vi "BeginService (reference).vi"(1 "In":i32) -> (0 "Out":i32)   [LabVIEW 2011]
doc: "Copyright (c) 2005, Kuan Chen\nAll rights reserved.\n\nRedistribution and use in source and binary forms, with or without modification, are permitted provided that the following conditions are met:\n\n * Redistributions of source code must retain the above copyright notice, this list of conditions and the following disclaimer.\n * Redistributions in binary form must reproduce the above copyright notice, this list of conditions and the following disclaimer in the documentation and/or other materials provided with the distribution.\n * Neither the name of the Kuan Chen nor the names of its contributors may be used to endorse or promote products derived from this software without specific prior written permission.\n\nTHIS SOFTWARE IS PROVIDED BY THE COPYRIGHT HOLDERS AND CONTRIBUTORS \"AS IS\" AND ANY EXPRESS OR IMPLIED WARRANTIES, INCLUDING, BUT NOT LIMITED TO, THE IMPLIED WARRANTIES OF MERCHANTABILITY AND FITNESS FOR A PARTICULAR PURPOSE ARE DISCLAIMED. IN NO EVENT SHALL THE COPYRIGHT OWNER OR CONTRIBUTORS BE LIABLE FOR ANY DIRECT, INDIRECT, INCIDENTAL, SPECIAL, EXEMPLARY, OR CONSEQUENTIAL DAMAGES (INCLUDING, BUT NOT LIMITED TO, PROCUREMENT OF SUBSTITUTE GOODS OR SERVICES; LOSS OF USE, DATA, OR PROFITS; OR BUSINESS INTERRUPTION) HOWEVER CAUSED AND ON ANY THEORY OF LIABILITY, WHETHER IN CONTRACT, STRICT LIABILITY, OR TORT (INCLUDING NEGLIGENCE OR OTHERWISE) ARISING IN ANY WAY OUT OF THE USE OF THIS SOFTWARE, EVEN IF ADVISED OF THE POSSIBILITY OF SUCH DAMAGE.\n\nWrites a \"line n\" line to C:\\temp\\output.txt once per second, where n is the nth second. Stops when StopOutputThread.vi is used."
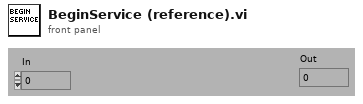
[diagram p1: front panel]
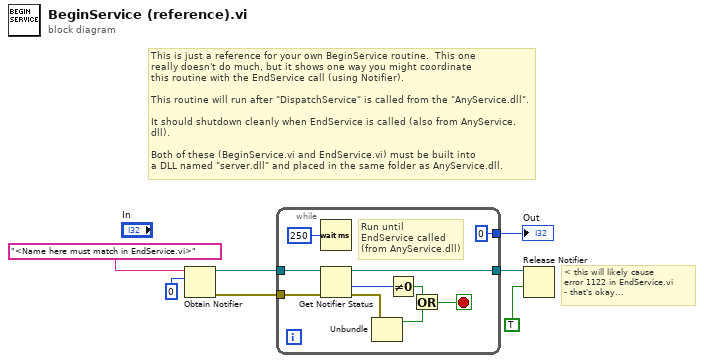
[diagram p0: block diagram]
diagram:
  # "This is just a reference for your own BeginService routine.  This one\nreally doesn't do much, but it shows one way you might coordinate\nthis routine with the EndService call (using Notifier).\n\nThis routine will run after \"DispatchService\" is called from the \"AnyService.dll\".\n\nIt should shutdown cleanly when EndService is called (also from AnyService.dll).\n\nBoth of these (BeginService.vi and EndService.vi) must be built into\na DLL named \"server.dll\" and placed in the same folder as AnyService.dll."
  # "< this will likely cause\nerror 1122 in EndService.vi\n- that's okay..."
  n1 = Obtain Notifier(name (unnamed)="<Name here must match in EndService.vi>", notification data type=0) -> (notifier out=w5:refnum<notifier>, error out=w4:errorcluster)  [unwired: 2 in, 1 out]
  n2 = while {
    tunnel: [0 ("Out")] -> w7
    tunnel: w5 -> [w16]
    tunnel: w4 -> [w15]
    tunnel: [w8] -> w2
    stop <- w11 stop-if-true
    # "Run until\nEndService called\n(from AnyService.dll)"
    n3 = Wait (ms)(milliseconds to wait=u32 250) -> ()  [unwired: 1 out]
    n4 = Get Notifier Status(notifier=w16, error in (no error)=w15) -> (notifier out=w8:refnum<notifier>, # waiting=w9:i32, error out=w13:errorcluster)  [unwired: 2 out]
    n5 = Unbundle(w13) -> ("status"=w12:bool)  [unwired: 2 out]
    n6 = Not Equal To 0?(x=w9) -> (x != 0?=w14:bool)
    n7 = Or(x=w14, y=w12) -> (x .or. y?=w11:bool)
  }
  "Out" <- w7
  n8 = Release Notifier(notifier=w2, force destroy? (F)=TRUE) -> ()  [unwired: 1 in, 3 out]
